vi "Y Axis Motor Speed Controller (1).vi"(1 "Speed Command (mm/s)":dbl) -> (0 "PWM  Frequency Command (Hz)":dbl)   [LabVIEW 2013]
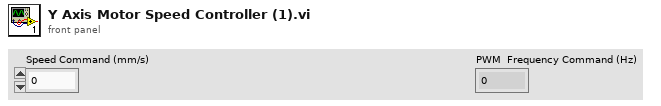
[diagram p1: front panel]
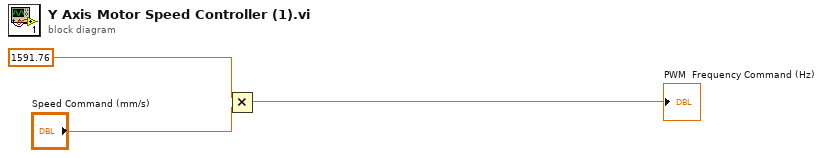
[diagram p0: block diagram]
diagram:
  n1 = Multiply(x=1591.76, y="Speed Command (mm/s)") -> (x*y=→"PWM  Frequency Command (Hz)":dbl)
